vi "Rubix Cube Array.vi"(7 "Rubix ref Array":refnum<vi>[][](array[refnum]), 8 "error in (no error)":errorcluster, 9 "Rubix Text Array in":string[][](array[string]), 10 "Face to act on":i32, 11 "Command":T2) -> (0 "error out(no error)":errorcluster, 1 "Axis":cluster{"X":sgl, "Y":sgl, "Z":sgl}, 2 "Rubix Array":T1[][](array[typedef]), 3 "Facets To move":T1[](array[typedef]), 5 "Rubix Text Array Out":string[][](array[string]))   [LabVIEW 2018]
uses:
  Cube Data Ops.ctl
  Rubix Array data type.ctl
  Rubix Global data type.ctl
  Rotate array command.ctl
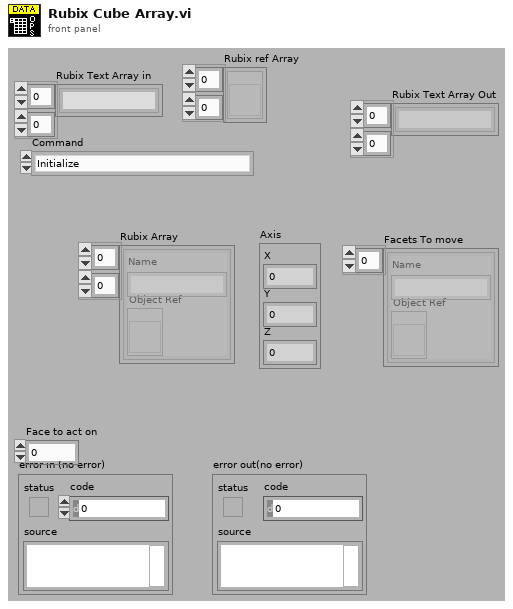
[diagram p1: front panel]
types:
  T1 = typedef "Rubix Array data type.ctl" = cluster{"Object Ref":refnum<vi>, "Name":string}
  T2 = typedef "Cube Data Ops.ctl" = enum16{"Initialize", "Set Rubix Ref Array", "Set Rubix Text Array", "Set Current Face", "Get Rubix Text Array", "Generate Rubix Array", "Get Rubix array", "Get Facets to move", "Randomize", "Top row left", "Top row right", "Middle row left", "Middle row right", "Bottom row left", "Bottom row right", "Left column up", "Left column down", "Middle column up", "Middle column down", "Right column up", "Right column down", "Face ccw", "Face cw"}
  T3 = typedef "Rubix Global data type.ctl" = cluster{"Rubix Text Array":string[][], "Face to act on":i32, "From":i32[], "Axis":cluster{"X":sgl, "Y":sgl, "Z":sgl}, "Rubix ref Array":refnum<vi>[][], "Rubix Array":T1[][], "Facets To move":T1[]}
  T4 = typedef "Rotate array command.ctl" = i32
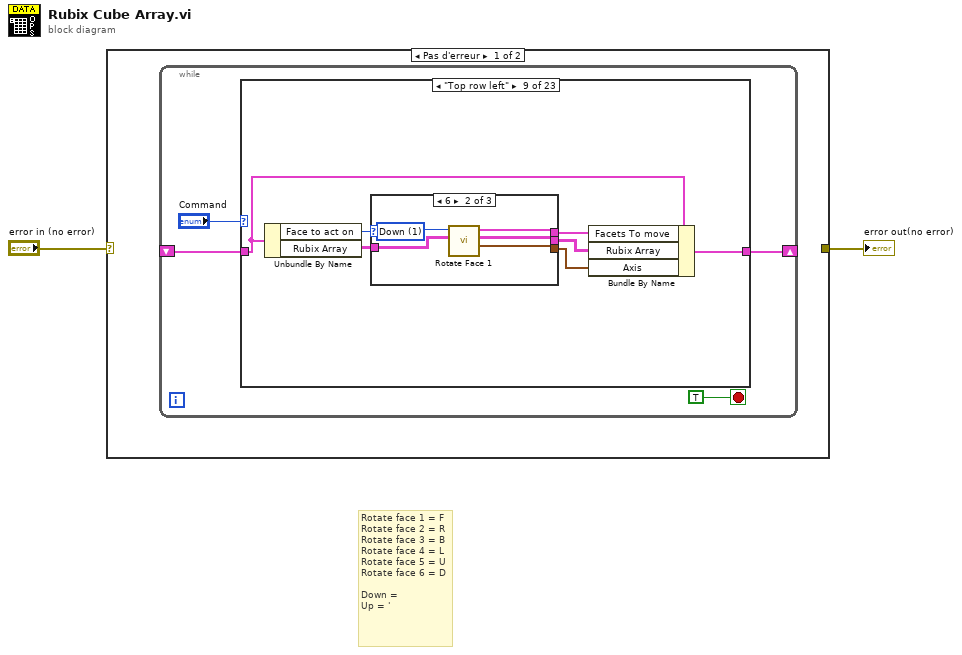
[diagram p0: block diagram]
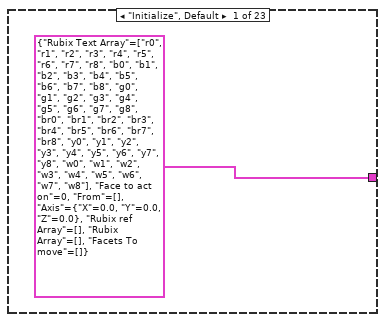
[diagram p2: hidden frame]
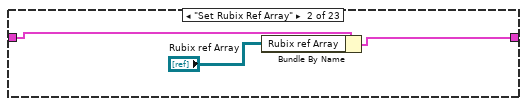
[diagram p3: hidden frame]
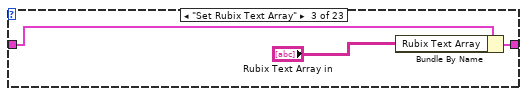
[diagram p4: hidden frame]
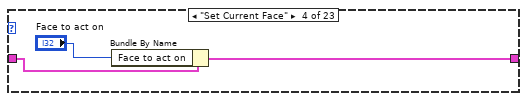
[diagram p5: hidden frame]
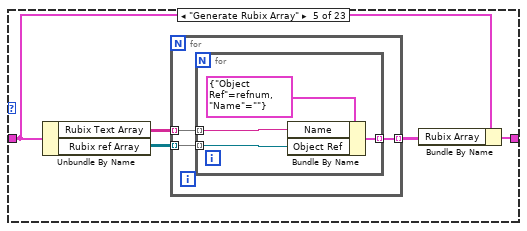
[diagram p6: hidden frame]
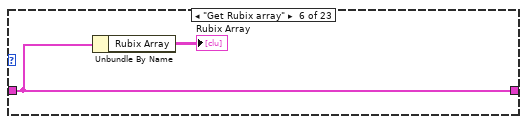
[diagram p7: hidden frame]
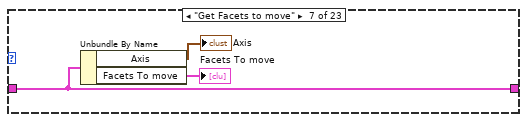
[diagram p8: hidden frame]
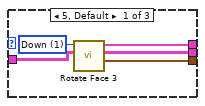
[diagram p10: hidden frame]
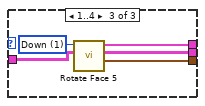
[diagram p11: hidden frame]
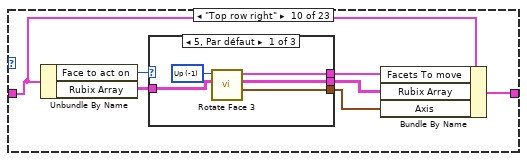
[diagram p12: hidden frame]
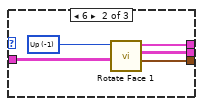
[diagram p13: hidden frame]
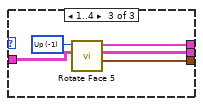
[diagram p14: hidden frame]
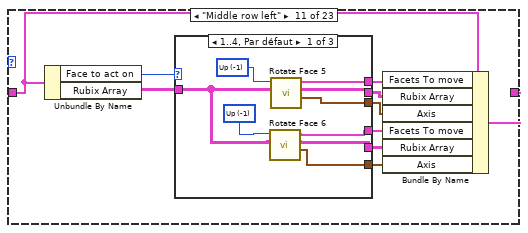
[diagram p15: hidden frame]
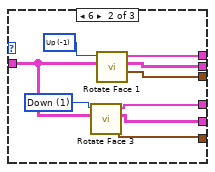
[diagram p16: hidden frame]
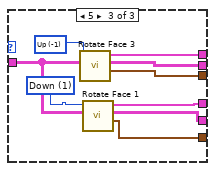
[diagram p17: hidden frame]
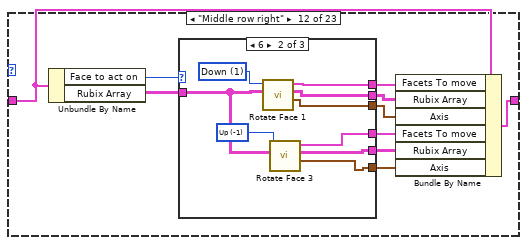
[diagram p18: hidden frame]
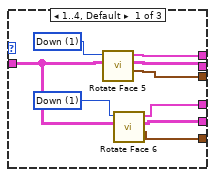
[diagram p19: hidden frame]
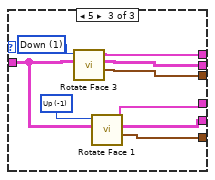
[diagram p20: hidden frame]
diagram:
  # "Rotate face 1 = F\nRotate face 2 = R\nRotate face 3 = B\nRotate face 4 = L\nRotate face 5 = U\nRotate face 6 = D\n\nDown = \nUp = '"
  n1 = case shown="Pas d'erreur" "error in (no error)" {
    selector: "error in (no error)" -> [_ w531]
    tunnel: [_ w531] -> w1
    frame No Error {
      n2 = while {
        shift-right: [w4] -> _
        shift-left: _ -> [w3]
        stop <- TRUE stop-if-true
        n3 = case shown="\"Top row left\"" "Command" {
          tunnel: [T3 {"Rubix Text Array"=[["r0", "r1", "r2", "r3", "r4", "r5", "r6", "r7", "r8"], ["b0", "b1", "b2", "b3", "b4", "b5", "b6", "b7", "b8"], ["g0", "g1", "g2", "g3", "g4", "g5", "g6", "g7", "g8"], ["br0", "br1", "br2", "br3", "br4", "br5", "br6", "br7", "br8"], ["y0", "y1", "y2", "y3", "y4", "y5", "y6", "y7", "y8"], ["w0", "w1", "w2", "w3", "w4", "w5", "w6", "w7", "w8"]], "Face to act on"=0, "From"=[], "Axis"={"X"=0.0, "Y"=0.0, "Z"=0.0}, "Rubix ref Array"=[], "Rubix Array"=[], "Facets To move"=[]} ("Cluster") w9 w13 w15 w17 w30 w33 w34 w41 w57 w88 w120 w158 w176 w201 w239 w280 w330 w381 w418 w455 w492 w529] -> w4
          tunnel: w3 -> [_ w10 w11 w16 w19 w30 w33 w34 w35 w58 w87 w119 w157 w175 w202 w238 w274 w329 w382 w419 w456 w493 w529]
          frame "Initialize", Default {
          }
          frame "Set Rubix Ref Array" {
            n4 = Bundle By Name(cluster=w10, "Rubix ref Array"="Rubix ref Array") -> (w9:T3)
          }
          frame "Set Rubix Text Array" {
            n5 = Bundle By Name(cluster=w11, "Rubix Text Array"="Rubix Text Array in") -> (w13:T3)
          }
          frame "Set Current Face" {
            n6 = Bundle By Name(cluster=w16, "Face to act on"="Face to act on") -> (w15:T3)
          }
          frame "Generate Rubix Array" {
            n7 = Unbundle By Name(w19) -> ("Rubix Text Array"=w21:string[][], "Rubix ref Array"=w20:refnum<vi>[][])
            n8 = for {
              tunnel: w21 -> [w24] mode=indexing
              tunnel: w20 -> [w23] mode=indexing
              tunnel: [w22] -> w18 mode=indexing
              n9 = for {
                tunnel: w24 -> [w27] mode=indexing
                tunnel: w23 -> [w25] mode=indexing
                tunnel: [w26] -> w22 mode=indexing
                n10 = Bundle By Name(cluster=T1 {"Object Ref"=refnum, "Name"=""} ("Rubix Array"), "Name"=w27, "Object Ref"=w25) -> (w26:T1)
              }
            }
            n11 = Bundle By Name(cluster=w19, "Rubix Array"=w18) -> (w17:T3)
          }
          frame "Get Rubix array" {
            n12 = Unbundle By Name(w30) -> ("Rubix Array"=→"Rubix Array":T1[][])
          }
          frame "Get Facets to move" {
            n13 = Unbundle By Name(w33) -> ("Axis"=→"Axis":cluster{"X":sgl, "Y":sgl, "Z":sgl}, "Facets To move"=→"Facets To move":T1[])
          }
          frame "Randomize" {
          }
          frame "Top row left" {
            n14 = Unbundle By Name(w35) -> ("Face to act on"=w40:i32, "Rubix Array"=w39:T1[][])
            n15 = case shown="6" w40 {
              tunnel: w39 -> [w43 w47 w55]
              tunnel: [w46 w51 w54] -> w38
              tunnel: [w45 w50 w53] -> w37
              tunnel: [w44 w49 w52] -> w36
              frame 5, Default {
                w42 = T4 1 items=["Up"=-1, "Down"=1] ("Command")
                n16 = call "Rotate Face 3.vi"("Pretransform Rubix Array"=w43, "Command"=w42) -> ("Axis"=w44:cluster{"X":sgl, "Y":sgl, "Z":sgl}, "Transform Rubix Array"=w45:T1[][], "Facets to move"=w46:T1[])  [unwired: 7 in]
              }
              frame 6 {
                w48 = T4 1 items=["Up"=-1, "Down"=1] ("Command")
                n17 = call "Rotate Face 1.vi"("Pretransform Rubix Array"=w47, "Command"=w48) -> ("Axis"=w49:cluster{"X":sgl, "Y":sgl, "Z":sgl}, "Transform Rubix Array"=w50:T1[][], "Facets to move"=w51:T1[])  [unwired: 7 in]
              }
              frame 1..4 {
                w56 = T4 1 items=["Up"=-1, "Down"=1] ("Command")
                n18 = call "Rotate Face 5.vi"("Pretransform Rubix Array"=w55, "Command"=w56) -> ("Axis"=w52:cluster{"X":sgl, "Y":sgl, "Z":sgl}, "Transform Rubix Array"=w53:T1[][], "Facets to move"=w54:T1[])  [unwired: 7 in]
              }
            }
            n19 = Bundle By Name(cluster=w35, "Facets To move"=w38, "Rubix Array"=w37, "Axis"=w36) -> (w41:T3)
          }
          frame "Top row right" {
            n20 = Unbundle By Name(w58) -> ("Face to act on"=w59:i32, "Rubix Array"=w60:T1[][])
            n21 = case shown="5, Par défaut" w59 {
              tunnel: w60 -> [w65 w73 w77]
              tunnel: [w68 w71 w76] -> w61
              tunnel: [w67 w70 w75] -> w62
              tunnel: [w66 w69 w74] -> w63
              frame 5, Default {
                w64 = T4 -1 items=["Up"=-1, "Down"=1] ("Command")
                n22 = call "Rotate Face 3.vi"("Pretransform Rubix Array"=w65, "Command"=w64) -> ("Axis"=w66:cluster{"X":sgl, "Y":sgl, "Z":sgl}, "Transform Rubix Array"=w67:T1[][], "Facets to move"=w68:T1[])  [unwired: 7 in]
              }
              frame 6 {
                w72 = T4 -1 items=["Up"=-1, "Down"=1] ("Command")
                n23 = call "Rotate Face 1.vi"("Pretransform Rubix Array"=w73, "Command"=w72) -> ("Axis"=w69:cluster{"X":sgl, "Y":sgl, "Z":sgl}, "Transform Rubix Array"=w70:T1[][], "Facets to move"=w71:T1[])  [unwired: 7 in]
              }
              frame 1..4 {
                w78 = T4 -1 items=["Up"=-1, "Down"=1] ("Command")
                n24 = call "Rotate Face 5.vi"("Pretransform Rubix Array"=w77, "Command"=w78) -> ("Axis"=w74:cluster{"X":sgl, "Y":sgl, "Z":sgl}, "Transform Rubix Array"=w75:T1[][], "Facets to move"=w76:T1[])  [unwired: 7 in]
              }
            }
            n25 = Bundle By Name(cluster=w58, "Facets To move"=w61, "Rubix Array"=w62, "Axis"=w63) -> (w57:T3)
          }
          frame "Middle row left" {
            n26 = Unbundle By Name(w87) -> ("Face to act on"=w86:i32, "Rubix Array"=w82:T1[][])
            n27 = case shown="1..4, Par défaut" w86 {
              tunnel: [w97 w100 w115] -> w85
              tunnel: [w95 w99 w114] -> w84
              tunnel: [w96 w98 w113] -> w83
              tunnel: w82 -> [w92 w102 w110]
              tunnel: [w91 w105 w109] -> w81
              tunnel: [w90 w104 w108] -> w80
              tunnel: [w89 w103 w107] -> w79
              frame 1..4, Default {
                w93 = T4 -1 items=["Up"=-1, "Down"=1] ("Command")
                w94 = T4 -1 items=["Up"=-1, "Down"=1] ("Command")
                n28 = call "Rotate Face 6.vi"("Pretransform Rubix Array"=w92, "Command"=w93) -> ("Axis"=w89:cluster{"X":sgl, "Y":sgl, "Z":sgl}, "Transform Rubix Array"=w90:T1[][], "Facets to move"=w91:T1[])  [unwired: 7 in]
                n29 = call "Rotate Face 5.vi"("Pretransform Rubix Array"=w92, "Command"=w94) -> ("Axis"=w96:cluster{"X":sgl, "Y":sgl, "Z":sgl}, "Transform Rubix Array"=w95:T1[][], "Facets to move"=w97:T1[])  [unwired: 7 in]
              }
              frame 6 {
                w106 = T4 1 items=["Up"=-1, "Down"=1] ("Command")
                w101 = T4 -1 items=["Up"=-1, "Down"=1] ("Command")
                n30 = call "Rotate Face 3.vi"("Pretransform Rubix Array"=w102, "Command"=w106) -> ("Axis"=w103:cluster{"X":sgl, "Y":sgl, "Z":sgl}, "Transform Rubix Array"=w104:T1[][], "Facets to move"=w105:T1[])  [unwired: 7 in]
                n31 = call "Rotate Face 1.vi"("Pretransform Rubix Array"=w102, "Command"=w101) -> ("Axis"=w98:cluster{"X":sgl, "Y":sgl, "Z":sgl}, "Transform Rubix Array"=w99:T1[][], "Facets to move"=w100:T1[])  [unwired: 7 in]
              }
              frame 5 {
                w111 = T4 1 items=["Up"=-1, "Down"=1] ("Command")
                w112 = T4 -1 items=["Up"=-1, "Down"=1] ("Command")
                n32 = call "Rotate Face 3.vi"("Pretransform Rubix Array"=w110, "Command"=w112) -> ("Axis"=w113:cluster{"X":sgl, "Y":sgl, "Z":sgl}, "Transform Rubix Array"=w114:T1[][], "Facets to move"=w115:T1[])  [unwired: 7 in]
                n33 = call "Rotate Face 1.vi"("Pretransform Rubix Array"=w110, "Command"=w111) -> ("Axis"=w107:cluster{"X":sgl, "Y":sgl, "Z":sgl}, "Transform Rubix Array"=w108:T1[][], "Facets to move"=w109:T1[])  [unwired: 7 in]
              }
            }
            n34 = Bundle By Name(cluster=w87, "Facets To move"=w85, "Rubix Array"=w84, "Axis"=w83, "Facets To move"=w81, "Rubix Array"=w80, "Axis"=w79) -> (w88:T3)
          }
          frame "Middle row right" {
            n35 = Unbundle By Name(w119) -> ("Face to act on"=w121:i32, "Rubix Array"=w125:T1[][])
            n36 = case shown="6" w121 {
              tunnel: [w134 w143 w152] -> w122
              tunnel: [w133 w142 w151] -> w123
              tunnel: [w132 w141 w150] -> w124
              tunnel: w125 -> [w129 w138 w147]
              tunnel: [w128 w137 w145] -> w118
              tunnel: [w127 w136 w144] -> w117
              tunnel: [w126 w135 w146] -> w116
              frame 1..4, Default {
                w130 = T4 1 items=["Up"=-1, "Down"=1] ("Command")
                w131 = T4 1 items=["Up"=-1, "Down"=1] ("Command")
                n37 = call "Rotate Face 5.vi"("Pretransform Rubix Array"=w129, "Command"=w131) -> ("Axis"=w132:cluster{"X":sgl, "Y":sgl, "Z":sgl}, "Transform Rubix Array"=w133:T1[][], "Facets to move"=w134:T1[])  [unwired: 7 in]
                n38 = call "Rotate Face 6.vi"("Pretransform Rubix Array"=w129, "Command"=w130) -> ("Axis"=w126:cluster{"X":sgl, "Y":sgl, "Z":sgl}, "Transform Rubix Array"=w127:T1[][], "Facets to move"=w128:T1[])  [unwired: 7 in]
              }
              frame 6 {
                w139 = T4 -1 items=["Up"=-1, "Down"=1] ("Command")
                w140 = T4 1 items=["Up"=-1, "Down"=1] ("Command")
                n39 = call "Rotate Face 1.vi"("Pretransform Rubix Array"=w138, "Command"=w140) -> ("Axis"=w141:cluster{"X":sgl, "Y":sgl, "Z":sgl}, "Transform Rubix Array"=w142:T1[][], "Facets to move"=w143:T1[])  [unwired: 7 in]
                n40 = call "Rotate Face 3.vi"("Pretransform Rubix Array"=w138, "Command"=w139) -> ("Axis"=w135:cluster{"X":sgl, "Y":sgl, "Z":sgl}, "Transform Rubix Array"=w136:T1[][], "Facets to move"=w137:T1[])  [unwired: 7 in]
              }
              frame 5 {
                w148 = T4 -1 items=["Up"=-1, "Down"=1] ("Command")
                w149 = T4 1 items=["Up"=-1, "Down"=1] ("Command")
                n41 = call "Rotate Face 3.vi"("Pretransform Rubix Array"=w147, "Command"=w149) -> ("Axis"=w150:cluster{"X":sgl, "Y":sgl, "Z":sgl}, "Transform Rubix Array"=w151:T1[][], "Facets to move"=w152:T1[])  [unwired: 7 in]
                n42 = call "Rotate Face 1.vi"("Pretransform Rubix Array"=w147, "Command"=w148) -> ("Axis"=w146:cluster{"X":sgl, "Y":sgl, "Z":sgl}, "Transform Rubix Array"=w144:T1[][], "Facets to move"=w145:T1[])  [unwired: 7 in]
              }
            }
            n43 = Bundle By Name(cluster=w119, "Facets To move"=w122, "Rubix Array"=w123, "Axis"=w124, "Facets To move"=w118, "Rubix Array"=w117, "Axis"=w116) -> (w120:T3)
          }
          frame "Bottom row left" {
            n44 = Unbundle By Name(w157) -> ("Face to act on"=w159:i32, "Rubix Array"=w153:T1[][])
            n45 = case shown="6" w159 {
              tunnel: [w164 w169 w174] -> w156
              tunnel: [w163 w167 w173] -> w155
              tunnel: [w162 w168 w172] -> w154
              tunnel: w153 -> [w161 w165 w170]
              frame 5, Default {
                w160 = T4 -1 items=["Up"=-1, "Down"=1] ("Command")
                n46 = call "Rotate Face 1.vi"("Pretransform Rubix Array"=w161, "Command"=w160) -> ("Axis"=w162:cluster{"X":sgl, "Y":sgl, "Z":sgl}, "Transform Rubix Array"=w163:T1[][], "Facets to move"=w164:T1[])  [unwired: 7 in]
              }
              frame 6 {
                w166 = T4 -1 items=["Up"=-1, "Down"=1] ("Command")
                n47 = call "Rotate Face 3.vi"("Pretransform Rubix Array"=w165, "Command"=w166) -> ("Axis"=w168:cluster{"X":sgl, "Y":sgl, "Z":sgl}, "Transform Rubix Array"=w167:T1[][], "Facets to move"=w169:T1[])  [unwired: 7 in]
              }
              frame 1..4 {
                w171 = T4 1 items=["Up"=-1, "Down"=1] ("Command")
                n48 = call "Rotate Face 6.vi"("Pretransform Rubix Array"=w170, "Command"=w171) -> ("Axis"=w172:cluster{"X":sgl, "Y":sgl, "Z":sgl}, "Transform Rubix Array"=w173:T1[][], "Facets to move"=w174:T1[])  [unwired: 7 in]
              }
            }
            n49 = Bundle By Name(cluster=w157, "Facets To move"=w156, "Rubix Array"=w155, "Axis"=w154) -> (w158:T3)
          }
          frame "Bottom row right" {
            n50 = Unbundle By Name(w175) -> ("Face to act on"=w177:i32, "Rubix Array"=w181:T1[][])
            n51 = case shown="1..4" w177 {
              tunnel: [w186 w191 w194] -> w178
              tunnel: [w185 w190 w193] -> w179
              tunnel: [w184 w189 w192] -> w180
              tunnel: w181 -> [w183 w188 w195]
              frame 5, Default {
                w182 = T4 1 items=["Up"=-1, "Down"=1] ("Command")
                n52 = call "Rotate Face 1.vi"("Pretransform Rubix Array"=w183, "Command"=w182) -> ("Axis"=w184:cluster{"X":sgl, "Y":sgl, "Z":sgl}, "Transform Rubix Array"=w185:T1[][], "Facets to move"=w186:T1[])  [unwired: 7 in]
              }
              frame 6 {
                w187 = T4 1 items=["Up"=-1, "Down"=1] ("Command")
                n53 = call "Rotate Face 3.vi"("Pretransform Rubix Array"=w188, "Command"=w187) -> ("Axis"=w189:cluster{"X":sgl, "Y":sgl, "Z":sgl}, "Transform Rubix Array"=w190:T1[][], "Facets to move"=w191:T1[])  [unwired: 7 in]
              }
              frame 1..4 {
                w196 = T4 -1 items=["Up"=-1, "Down"=1] ("Command")
                n54 = call "Rotate Face 6.vi"("Pretransform Rubix Array"=w195, "Command"=w196) -> ("Axis"=w192:cluster{"X":sgl, "Y":sgl, "Z":sgl}, "Transform Rubix Array"=w193:T1[][], "Facets to move"=w194:T1[])  [unwired: 7 in]
              }
            }
            n55 = Bundle By Name(cluster=w175, "Facets To move"=w178, "Rubix Array"=w179, "Axis"=w180) -> (w176:T3)
          }
          frame "Left column up" {
            n56 = Unbundle By Name(w202) -> ("Face to act on"=w203:i32, "Rubix Array"=w198:T1[][])
            n57 = case shown="6" w203 {
              tunnel: [w207 w210 w216 w221 w226 w232] -> w200
              tunnel: [w208 w212 w218 w223 w228 w233] -> w197
              tunnel: [w206 w211 w217 w222 w227 w231] -> w199
              tunnel: w198 -> [w205 w209 w215 w220 w225 w230]
              frame 1 {
                w204 = T4 -1 items=["Up"=-1, "Down"=1] ("Command")
                n58 = call "Rotate Face 4.vi"("Pretransform Rubix Array"=w205, "Command"=w204) -> ("Axis"=w206:cluster{"X":sgl, "Y":sgl, "Z":sgl}, "Transform Rubix Array"=w207:T1[][], "Facets to move"=w208:T1[])  [unwired: 7 in]
              }
              frame 2 {
                w213 = T4 -1 items=["Up"=-1, "Down"=1] ("Command")
                n59 = call "Rotate Face 1.vi"("Pretransform Rubix Array"=w209, "Command"=w213) -> ("Axis"=w211:cluster{"X":sgl, "Y":sgl, "Z":sgl}, "Transform Rubix Array"=w210:T1[][], "Facets to move"=w212:T1[])  [unwired: 7 in]
              }
              frame 3 {
                w214 = T4 -1 items=["Up"=-1, "Down"=1] ("Command")
                n60 = call "Rotate Face 2.vi"("Pretransform Rubix Array"=w215, "Command"=w214) -> ("Axis"=w217:cluster{"X":sgl, "Y":sgl, "Z":sgl}, "Transform Rubix Array"=w216:T1[][], "Facets to move"=w218:T1[])  [unwired: 7 in]
              }
              frame 4 {
                w219 = T4 -1 items=["Up"=-1, "Down"=1] ("Command")
                n61 = call "Rotate Face 3.vi"("Pretransform Rubix Array"=w220, "Command"=w219) -> ("Axis"=w222:cluster{"X":sgl, "Y":sgl, "Z":sgl}, "Transform Rubix Array"=w221:T1[][], "Facets to move"=w223:T1[])  [unwired: 7 in]
              }
              frame 5, Default {
                w224 = T4 -1 items=["Up"=-1, "Down"=1] ("Command")
                n62 = call "Rotate Face 4.vi"("Pretransform Rubix Array"=w225, "Command"=w224) -> ("Axis"=w227:cluster{"X":sgl, "Y":sgl, "Z":sgl}, "Transform Rubix Array"=w226:T1[][], "Facets to move"=w228:T1[])  [unwired: 7 in]
              }
              frame 6 {
                w229 = T4 -1 items=["Up"=-1, "Down"=1] ("Command")
                n63 = call "Rotate Face 4.vi"("Pretransform Rubix Array"=w230, "Command"=w229) -> ("Axis"=w231:cluster{"X":sgl, "Y":sgl, "Z":sgl}, "Transform Rubix Array"=w232:T1[][], "Facets to move"=w233:T1[])  [unwired: 7 in]
              }
            }
            n64 = Bundle By Name(cluster=w202, "Facets To move"=w197, "Rubix Array"=w200, "Axis"=w199) -> (w201:T3)
          }
          frame "Left column down" {
            n65 = Unbundle By Name(w238) -> ("Face to act on"=w237:i32, "Rubix Array"=w240:T1[][])
            n66 = case shown="6" w237 {
              tunnel: w240 -> [w241 w247 w252 w259 w262 w267]
              tunnel: [w244 w250 w255 w258 w265 w270] -> w236
              tunnel: [w243 w249 w254 w257 w264 w269] -> w235
              tunnel: [w242 w248 w253 w256 w263 w268] -> w234
              frame 2, Default {
                w245 = T4 1 items=["Up"=-1, "Down"=1] ("Command")
                n67 = call "Rotate Face 1.vi"("Pretransform Rubix Array"=w241, "Command"=w245) -> ("Axis"=w242:cluster{"X":sgl, "Y":sgl, "Z":sgl}, "Transform Rubix Array"=w243:T1[][], "Facets to move"=w244:T1[])  [unwired: 7 in]
              }
              frame 3 {
                w246 = T4 1 items=["Up"=-1, "Down"=1] ("Command")
                n68 = call "Rotate Face 2.vi"("Pretransform Rubix Array"=w247, "Command"=w246) -> ("Axis"=w248:cluster{"X":sgl, "Y":sgl, "Z":sgl}, "Transform Rubix Array"=w249:T1[][], "Facets to move"=w250:T1[])  [unwired: 7 in]
              }
              frame 4 {
                w251 = T4 1 items=["Up"=-1, "Down"=1] ("Command")
                n69 = call "Rotate Face 3.vi"("Pretransform Rubix Array"=w252, "Command"=w251) -> ("Axis"=w253:cluster{"X":sgl, "Y":sgl, "Z":sgl}, "Transform Rubix Array"=w254:T1[][], "Facets to move"=w255:T1[])  [unwired: 7 in]
              }
              frame 5 {
                w260 = T4 1 items=["Up"=-1, "Down"=1] ("Command")
                n70 = call "Rotate Face 4.vi"("Pretransform Rubix Array"=w259, "Command"=w260) -> ("Axis"=w256:cluster{"X":sgl, "Y":sgl, "Z":sgl}, "Transform Rubix Array"=w257:T1[][], "Facets to move"=w258:T1[])  [unwired: 7 in]
              }
              frame 6 {
                w261 = T4 1 items=["Up"=-1, "Down"=1] ("Command")
                n71 = call "Rotate Face 4.vi"("Pretransform Rubix Array"=w262, "Command"=w261) -> ("Axis"=w263:cluster{"X":sgl, "Y":sgl, "Z":sgl}, "Transform Rubix Array"=w264:T1[][], "Facets to move"=w265:T1[])  [unwired: 7 in]
              }
              frame 1 {
                w266 = T4 1 items=["Up"=-1, "Down"=1] ("Command")
                n72 = call "Rotate Face 4.vi"("Pretransform Rubix Array"=w267, "Command"=w266) -> ("Axis"=w268:cluster{"X":sgl, "Y":sgl, "Z":sgl}, "Transform Rubix Array"=w269:T1[][], "Facets to move"=w270:T1[])  [unwired: 7 in]
              }
            }
            n73 = Bundle By Name(cluster=w238, "Facets To move"=w236, "Rubix Array"=w235, "Axis"=w234) -> (w239:T3)
          }
          frame "Middle column up" {
            n74 = Unbundle By Name(w274) -> ("Face to act on"=w279:i32, "Rubix Array"=w278:T1[][])
            n75 = case shown="6" w279 {
              tunnel: w278 -> [w284 w293 w302 w311 w320]
              tunnel: [w287 w296 w305 w314 w323] -> w277
              tunnel: [w288 w297 w306 w315 w324] -> w276
              tunnel: [w286 w295 w304 w313 w322] -> w275
              tunnel: [w283 w292 w301 w310 w319] -> w273
              tunnel: [w282 w291 w300 w309 w318] -> w272
              tunnel: [w281 w290 w299 w308 w317] -> w271
              frame 1, 5 {
                w285 = T4 -1 items=["Up"=-1, "Down"=1] ("Command")
                w289 = T4 1 items=["Up"=-1, "Down"=1] ("Command")
                n76 = call "Rotate Face 4.vi"("Pretransform Rubix Array"=w284, "Command"=w289) -> ("Axis"=w286:cluster{"X":sgl, "Y":sgl, "Z":sgl}, "Transform Rubix Array"=w287:T1[][], "Facets to move"=w288:T1[])  [unwired: 7 in]
                n77 = call "Rotate Face 2.vi"("Pretransform Rubix Array"=w284, "Command"=w285) -> ("Axis"=w281:cluster{"X":sgl, "Y":sgl, "Z":sgl}, "Transform Rubix Array"=w282:T1[][], "Facets to move"=w283:T1[])  [unwired: 7 in]
              }
              frame 2, Default {
                w294 = T4 -1 items=["Up"=-1, "Down"=1] ("Command")
                w298 = T4 1 items=["Up"=-1, "Down"=1] ("Command")
                n78 = call "Rotate Face 3.vi"("Pretransform Rubix Array"=w293, "Command"=w294) -> ("Axis"=w290:cluster{"X":sgl, "Y":sgl, "Z":sgl}, "Transform Rubix Array"=w291:T1[][], "Facets to move"=w292:T1[])  [unwired: 7 in]
                n79 = call "Rotate Face 1.vi"("Pretransform Rubix Array"=w293, "Command"=w298) -> ("Axis"=w295:cluster{"X":sgl, "Y":sgl, "Z":sgl}, "Transform Rubix Array"=w296:T1[][], "Facets to move"=w297:T1[])  [unwired: 7 in]
              }
              frame 3 {
                w303 = T4 -1 items=["Up"=-1, "Down"=1] ("Command")
                w307 = T4 1 items=["Up"=-1, "Down"=1] ("Command")
                n80 = call "Rotate Face 4.vi"("Pretransform Rubix Array"=w302, "Command"=w303) -> ("Axis"=w299:cluster{"X":sgl, "Y":sgl, "Z":sgl}, "Transform Rubix Array"=w300:T1[][], "Facets to move"=w301:T1[])  [unwired: 7 in]
                n81 = call "Rotate Face 2.vi"("Pretransform Rubix Array"=w302, "Command"=w307) -> ("Axis"=w304:cluster{"X":sgl, "Y":sgl, "Z":sgl}, "Transform Rubix Array"=w305:T1[][], "Facets to move"=w306:T1[])  [unwired: 7 in]
              }
              frame 6 {
                w312 = T4 -1 items=["Up"=-1, "Down"=1] ("Command")
                w316 = T4 1 items=["Up"=-1, "Down"=1] ("Command")
                n82 = call "Rotate Face 2.vi"("Pretransform Rubix Array"=w311, "Command"=w312) -> ("Axis"=w308:cluster{"X":sgl, "Y":sgl, "Z":sgl}, "Transform Rubix Array"=w309:T1[][], "Facets to move"=w310:T1[])  [unwired: 7 in]
                n83 = call "Rotate Face 4.vi"("Pretransform Rubix Array"=w311, "Command"=w316) -> ("Axis"=w313:cluster{"X":sgl, "Y":sgl, "Z":sgl}, "Transform Rubix Array"=w314:T1[][], "Facets to move"=w315:T1[])  [unwired: 7 in]
              }
              frame 4 {
                w321 = T4 -1 items=["Up"=-1, "Down"=1] ("Command")
                w325 = T4 1 items=["Up"=-1, "Down"=1] ("Command")
                n84 = call "Rotate Face 1.vi"("Pretransform Rubix Array"=w320, "Command"=w321) -> ("Axis"=w317:cluster{"X":sgl, "Y":sgl, "Z":sgl}, "Transform Rubix Array"=w318:T1[][], "Facets to move"=w319:T1[])  [unwired: 7 in]
                n85 = call "Rotate Face 3.vi"("Pretransform Rubix Array"=w320, "Command"=w325) -> ("Axis"=w322:cluster{"X":sgl, "Y":sgl, "Z":sgl}, "Transform Rubix Array"=w323:T1[][], "Facets to move"=w324:T1[])  [unwired: 7 in]
              }
            }
            n86 = Bundle By Name(cluster=w274, "Facets To move"=w276, "Rubix Array"=w277, "Axis"=w275, "Facets To move"=w273, "Rubix Array"=w272, "Axis"=w271) -> (w280:T3)
          }
          frame "Middle column down" {
            n87 = Unbundle By Name(w329) -> ("Face to act on"=w331:i32, "Rubix Array"=w332:T1[][])
            n88 = case shown="6" w331 {
              tunnel: w332 -> [w339 w348 w354 w366 w375]
              tunnel: [w342 w351 w360 w369 w378] -> w333
              tunnel: [w343 w352 w361 w370 w379] -> w334
              tunnel: [w341 w350 w359 w368 w377] -> w335
              tunnel: [w338 w345 w356 w363 w372] -> w328
              tunnel: [w337 w346 w357 w364 w373] -> w327
              tunnel: [w336 w347 w358 w365 w374] -> w326
              frame 1, 5 {
                w340 = T4 1 items=["Up"=-1, "Down"=1] ("Command")
                w344 = T4 -1 items=["Up"=-1, "Down"=1] ("Command")
                n89 = call "Rotate Face 2.vi"("Pretransform Rubix Array"=w339, "Command"=w340) -> ("Axis"=w338:cluster{"X":sgl, "Y":sgl, "Z":sgl}, "Transform Rubix Array"=w337:T1[][], "Facets to move"=w336:T1[])  [unwired: 7 in]
                n90 = call "Rotate Face 4.vi"("Pretransform Rubix Array"=w339, "Command"=w344) -> ("Axis"=w341:cluster{"X":sgl, "Y":sgl, "Z":sgl}, "Transform Rubix Array"=w342:T1[][], "Facets to move"=w343:T1[])  [unwired: 7 in]
              }
              frame 2, Default {
                w349 = T4 1 items=["Up"=-1, "Down"=1] ("Command")
                w353 = T4 -1 items=["Up"=-1, "Down"=1] ("Command")
                n91 = call "Rotate Face 3.vi"("Pretransform Rubix Array"=w348, "Command"=w349) -> ("Axis"=w345:cluster{"X":sgl, "Y":sgl, "Z":sgl}, "Transform Rubix Array"=w346:T1[][], "Facets to move"=w347:T1[])  [unwired: 7 in]
                n92 = call "Rotate Face 1.vi"("Pretransform Rubix Array"=w348, "Command"=w353) -> ("Axis"=w350:cluster{"X":sgl, "Y":sgl, "Z":sgl}, "Transform Rubix Array"=w351:T1[][], "Facets to move"=w352:T1[])  [unwired: 7 in]
              }
              frame 3 {
                w355 = T4 1 items=["Up"=-1, "Down"=1] ("Command")
                w362 = T4 -1 items=["Up"=-1, "Down"=1] ("Command")
                n93 = call "Rotate Face 4.vi"("Pretransform Rubix Array"=w354, "Command"=w355) -> ("Axis"=w356:cluster{"X":sgl, "Y":sgl, "Z":sgl}, "Transform Rubix Array"=w357:T1[][], "Facets to move"=w358:T1[])  [unwired: 7 in]
                n94 = call "Rotate Face 2.vi"("Pretransform Rubix Array"=w354, "Command"=w362) -> ("Axis"=w359:cluster{"X":sgl, "Y":sgl, "Z":sgl}, "Transform Rubix Array"=w360:T1[][], "Facets to move"=w361:T1[])  [unwired: 7 in]
              }
              frame 6 {
                w367 = T4 1 items=["Up"=-1, "Down"=1] ("Command")
                w371 = T4 -1 items=["Up"=-1, "Down"=1] ("Command")
                n95 = call "Rotate Face 4.vi"("Pretransform Rubix Array"=w366, "Command"=w371) -> ("Axis"=w368:cluster{"X":sgl, "Y":sgl, "Z":sgl}, "Transform Rubix Array"=w369:T1[][], "Facets to move"=w370:T1[])  [unwired: 7 in]
                n96 = call "Rotate Face 2.vi"("Pretransform Rubix Array"=w366, "Command"=w367) -> ("Axis"=w363:cluster{"X":sgl, "Y":sgl, "Z":sgl}, "Transform Rubix Array"=w364:T1[][], "Facets to move"=w365:T1[])  [unwired: 7 in]
              }
              frame 4 {
                w376 = T4 1 items=["Up"=-1, "Down"=1] ("Command")
                w380 = T4 -1 items=["Up"=-1, "Down"=1] ("Command")
                n97 = call "Rotate Face 1.vi"("Pretransform Rubix Array"=w375, "Command"=w376) -> ("Axis"=w372:cluster{"X":sgl, "Y":sgl, "Z":sgl}, "Transform Rubix Array"=w373:T1[][], "Facets to move"=w374:T1[])  [unwired: 7 in]
                n98 = call "Rotate Face 3.vi"("Pretransform Rubix Array"=w375, "Command"=w380) -> ("Axis"=w377:cluster{"X":sgl, "Y":sgl, "Z":sgl}, "Transform Rubix Array"=w378:T1[][], "Facets to move"=w379:T1[])  [unwired: 7 in]
              }
            }
            n99 = Bundle By Name(cluster=w329, "Facets To move"=w334, "Rubix Array"=w333, "Axis"=w335, "Facets To move"=w326, "Rubix Array"=w327, "Axis"=w328) -> (w330:T3)
          }
          frame "Right column up" {
            n100 = Unbundle By Name(w382) -> ("Face to act on"=w383:i32, "Rubix Array"=w386:T1[][])
            n101 = case shown="6" w383 {
              tunnel: [w391 w396 w401 w406 w411 w414] -> w384
              tunnel: [w392 w397 w402 w407 w412 w415] -> w387
              tunnel: [w390 w395 w400 w405 w410 w413] -> w385
              tunnel: w386 -> [w388 w394 w398 w404 w409 w416]
              frame 1 {
                w389 = T4 1 items=["Up"=-1, "Down"=1] ("Command")
                n102 = call "Rotate Face 2.vi"("Pretransform Rubix Array"=w388, "Command"=w389) -> ("Axis"=w390:cluster{"X":sgl, "Y":sgl, "Z":sgl}, "Transform Rubix Array"=w391:T1[][], "Facets to move"=w392:T1[])  [unwired: 7 in]
              }
              frame 2 {
                w393 = T4 1 items=["Up"=-1, "Down"=1] ("Command")
                n103 = call "Rotate Face 3.vi"("Pretransform Rubix Array"=w394, "Command"=w393) -> ("Axis"=w395:cluster{"X":sgl, "Y":sgl, "Z":sgl}, "Transform Rubix Array"=w396:T1[][], "Facets to move"=w397:T1[])  [unwired: 7 in]
              }
              frame 3 {
                w399 = T4 1 items=["Up"=-1, "Down"=1] ("Command")
                n104 = call "Rotate Face 4.vi"("Pretransform Rubix Array"=w398, "Command"=w399) -> ("Axis"=w400:cluster{"X":sgl, "Y":sgl, "Z":sgl}, "Transform Rubix Array"=w401:T1[][], "Facets to move"=w402:T1[])  [unwired: 7 in]
              }
              frame 4 {
                w403 = T4 1 items=["Up"=-1, "Down"=1] ("Command")
                n105 = call "Rotate Face 1.vi"("Pretransform Rubix Array"=w404, "Command"=w403) -> ("Axis"=w405:cluster{"X":sgl, "Y":sgl, "Z":sgl}, "Transform Rubix Array"=w406:T1[][], "Facets to move"=w407:T1[])  [unwired: 7 in]
              }
              frame 5, Default {
                w408 = T4 1 items=["Up"=-1, "Down"=1] ("Command")
                n106 = call "Rotate Face 2.vi"("Pretransform Rubix Array"=w409, "Command"=w408) -> ("Axis"=w410:cluster{"X":sgl, "Y":sgl, "Z":sgl}, "Transform Rubix Array"=w411:T1[][], "Facets to move"=w412:T1[])  [unwired: 7 in]
              }
              frame 6 {
                w417 = T4 1 items=["Up"=-1, "Down"=1] ("Command")
                n107 = call "Rotate Face 2.vi"("Pretransform Rubix Array"=w416, "Command"=w417) -> ("Axis"=w413:cluster{"X":sgl, "Y":sgl, "Z":sgl}, "Transform Rubix Array"=w414:T1[][], "Facets to move"=w415:T1[])  [unwired: 7 in]
              }
            }
            n108 = Bundle By Name(cluster=w382, "Facets To move"=w387, "Rubix Array"=w384, "Axis"=w385) -> (w381:T3)
          }
          frame "Right column down" {
            n109 = Unbundle By Name(w419) -> ("Face to act on"=w424:i32, "Rubix Array"=w421:T1[][])
            n110 = case shown="6" w424 {
              tunnel: [w428 w433 w438 w443 w448 w453] -> w423
              tunnel: [w429 w434 w439 w444 w449 w454] -> w420
              tunnel: [w427 w432 w437 w442 w447 w452] -> w422
              tunnel: w421 -> [w425 w431 w435 w441 w446 w451]
              frame 1 {
                w426 = T4 -1 items=["Up"=-1, "Down"=1] ("Command")
                n111 = call "Rotate Face 2.vi"("Pretransform Rubix Array"=w425, "Command"=w426) -> ("Axis"=w427:cluster{"X":sgl, "Y":sgl, "Z":sgl}, "Transform Rubix Array"=w428:T1[][], "Facets to move"=w429:T1[])  [unwired: 7 in]
              }
              frame 2 {
                w430 = T4 -1 items=["Up"=-1, "Down"=1] ("Command")
                n112 = call "Rotate Face 3.vi"("Pretransform Rubix Array"=w431, "Command"=w430) -> ("Axis"=w432:cluster{"X":sgl, "Y":sgl, "Z":sgl}, "Transform Rubix Array"=w433:T1[][], "Facets to move"=w434:T1[])  [unwired: 7 in]
              }
              frame 3 {
                w436 = T4 -1 items=["Up"=-1, "Down"=1] ("Command")
                n113 = call "Rotate Face 4.vi"("Pretransform Rubix Array"=w435, "Command"=w436) -> ("Axis"=w437:cluster{"X":sgl, "Y":sgl, "Z":sgl}, "Transform Rubix Array"=w438:T1[][], "Facets to move"=w439:T1[])  [unwired: 7 in]
              }
              frame 4 {
                w440 = T4 -1 items=["Up"=-1, "Down"=1] ("Command")
                n114 = call "Rotate Face 1.vi"("Pretransform Rubix Array"=w441, "Command"=w440) -> ("Axis"=w442:cluster{"X":sgl, "Y":sgl, "Z":sgl}, "Transform Rubix Array"=w443:T1[][], "Facets to move"=w444:T1[])  [unwired: 7 in]
              }
              frame 5, Default {
                w445 = T4 -1 items=["Up"=-1, "Down"=1] ("Command")
                n115 = call "Rotate Face 2.vi"("Pretransform Rubix Array"=w446, "Command"=w445) -> ("Axis"=w447:cluster{"X":sgl, "Y":sgl, "Z":sgl}, "Transform Rubix Array"=w448:T1[][], "Facets to move"=w449:T1[])  [unwired: 7 in]
              }
              frame 6 {
                w450 = T4 -1 items=["Up"=-1, "Down"=1] ("Command")
                n116 = call "Rotate Face 2.vi"("Pretransform Rubix Array"=w451, "Command"=w450) -> ("Axis"=w452:cluster{"X":sgl, "Y":sgl, "Z":sgl}, "Transform Rubix Array"=w453:T1[][], "Facets to move"=w454:T1[])  [unwired: 7 in]
              }
            }
            n117 = Bundle By Name(cluster=w419, "Facets To move"=w420, "Rubix Array"=w423, "Axis"=w422) -> (w418:T3)
          }
          frame "Face ccw" {
            n118 = Unbundle By Name(w456) -> ("Face to act on"=w457:i32, "Rubix Array"=w460:T1[][])
            n119 = case shown="1" w457 {
              tunnel: [w465 w470 w475 w480 w485 w490] -> w458
              tunnel: [w466 w471 w476 w481 w486 w491] -> w461
              tunnel: [w464 w469 w474 w479 w484 w489] -> w459
              tunnel: w460 -> [w463 w467 w472 w478 w483 w488]
              frame 1 {
                w462 = T4 -1 items=["Up"=-1, "Down"=1] ("Command")
                n120 = call "Rotate Face 1.vi"("Pretransform Rubix Array"=w463, "Command"=w462) -> ("Axis"=w464:cluster{"X":sgl, "Y":sgl, "Z":sgl}, "Transform Rubix Array"=w465:T1[][], "Facets to move"=w466:T1[])  [unwired: 7 in]
              }
              frame 2 {
                w468 = T4 -1 items=["Up"=-1, "Down"=1] ("Command")
                n121 = call "Rotate Face 2.vi"("Pretransform Rubix Array"=w467, "Command"=w468) -> ("Axis"=w469:cluster{"X":sgl, "Y":sgl, "Z":sgl}, "Transform Rubix Array"=w470:T1[][], "Facets to move"=w471:T1[])  [unwired: 7 in]
              }
              frame 3 {
                w473 = T4 -1 items=["Up"=-1, "Down"=1] ("Command")
                n122 = call "Rotate Face 3.vi"("Pretransform Rubix Array"=w472, "Command"=w473) -> ("Axis"=w474:cluster{"X":sgl, "Y":sgl, "Z":sgl}, "Transform Rubix Array"=w475:T1[][], "Facets to move"=w476:T1[])  [unwired: 7 in]
              }
              frame 4 {
                w477 = T4 -1 items=["Up"=-1, "Down"=1] ("Command")
                n123 = call "Rotate Face 4.vi"("Pretransform Rubix Array"=w478, "Command"=w477) -> ("Axis"=w479:cluster{"X":sgl, "Y":sgl, "Z":sgl}, "Transform Rubix Array"=w480:T1[][], "Facets to move"=w481:T1[])  [unwired: 7 in]
              }
              frame 5, Default {
                w482 = T4 -1 items=["Up"=-1, "Down"=1] ("Command")
                n124 = call "Rotate Face 5.vi"("Pretransform Rubix Array"=w483, "Command"=w482) -> ("Axis"=w484:cluster{"X":sgl, "Y":sgl, "Z":sgl}, "Transform Rubix Array"=w485:T1[][], "Facets to move"=w486:T1[])  [unwired: 7 in]
              }
              frame 6 {
                w487 = T4 1 items=["Up"=-1, "Down"=1] ("Command")
                n125 = call "Rotate Face 6.vi"("Pretransform Rubix Array"=w488, "Command"=w487) -> ("Axis"=w489:cluster{"X":sgl, "Y":sgl, "Z":sgl}, "Transform Rubix Array"=w490:T1[][], "Facets to move"=w491:T1[])  [unwired: 7 in]
              }
            }
            n126 = Bundle By Name(cluster=w456, "Facets To move"=w461, "Rubix Array"=w458, "Axis"=w459) -> (w455:T3)
          }
          frame "Face cw" {
            n127 = Unbundle By Name(w493) -> ("Face to act on"=w498:i32, "Rubix Array"=w495:T1[][])
            n128 = case shown="1" w498 {
              tunnel: [w502 w507 w512 w517 w522 w527] -> w497
              tunnel: [w503 w508 w513 w518 w523 w528] -> w494
              tunnel: [w501 w506 w511 w516 w521 w526] -> w496
              tunnel: w495 -> [w500 w504 w509 w515 w520 w525]
              frame 1 {
                w499 = T4 1 items=["Up"=-1, "Down"=1] ("Command")
                n129 = call "Rotate Face 1.vi"("Pretransform Rubix Array"=w500, "Command"=w499) -> ("Axis"=w501:cluster{"X":sgl, "Y":sgl, "Z":sgl}, "Transform Rubix Array"=w502:T1[][], "Facets to move"=w503:T1[])  [unwired: 7 in]
              }
              frame 2 {
                w505 = T4 1 items=["Up"=-1, "Down"=1] ("Command")
                n130 = call "Rotate Face 2.vi"("Pretransform Rubix Array"=w504, "Command"=w505) -> ("Axis"=w506:cluster{"X":sgl, "Y":sgl, "Z":sgl}, "Transform Rubix Array"=w507:T1[][], "Facets to move"=w508:T1[])  [unwired: 7 in]
              }
              frame 3 {
                w510 = T4 1 items=["Up"=-1, "Down"=1] ("Command")
                n131 = call "Rotate Face 3.vi"("Pretransform Rubix Array"=w509, "Command"=w510) -> ("Axis"=w511:cluster{"X":sgl, "Y":sgl, "Z":sgl}, "Transform Rubix Array"=w512:T1[][], "Facets to move"=w513:T1[])  [unwired: 7 in]
              }
              frame 4 {
                w514 = T4 1 items=["Up"=-1, "Down"=1] ("Command")
                n132 = call "Rotate Face 4.vi"("Pretransform Rubix Array"=w515, "Command"=w514) -> ("Axis"=w516:cluster{"X":sgl, "Y":sgl, "Z":sgl}, "Transform Rubix Array"=w517:T1[][], "Facets to move"=w518:T1[])  [unwired: 7 in]
              }
              frame 5, Default {
                w519 = T4 1 items=["Up"=-1, "Down"=1] ("Command")
                n133 = call "Rotate Face 5.vi"("Pretransform Rubix Array"=w520, "Command"=w519) -> ("Axis"=w521:cluster{"X":sgl, "Y":sgl, "Z":sgl}, "Transform Rubix Array"=w522:T1[][], "Facets to move"=w523:T1[])  [unwired: 7 in]
              }
              frame 6 {
                w524 = T4 -1 items=["Up"=-1, "Down"=1] ("Command")
                n134 = call "Rotate Face 6.vi"("Pretransform Rubix Array"=w525, "Command"=w524) -> ("Axis"=w526:cluster{"X":sgl, "Y":sgl, "Z":sgl}, "Transform Rubix Array"=w527:T1[][], "Facets to move"=w528:T1[])  [unwired: 7 in]
              }
            }
            n135 = Bundle By Name(cluster=w493, "Facets To move"=w494, "Rubix Array"=w497, "Axis"=w496) -> (w492:T3)
          }
          frame "Get Rubix Text Array" {
            n136 = Unbundle By Name(w529) -> ("Rubix Text Array"=→"Rubix Text Array Out":string[][])
          }
        }
      }
    }
    frame Error {
    }
  }
  "error out(no error)" <- w1
